vi "Shot.vi"(0 "CCD monitor in":refnum<class "CCD monitor.lvclass">, 5 "Numeric":u32, 7 "PhotoPath":path, 9 "Value":enum16{"1X1", "2X2"}(ring), 11 "error in (no error)":errorcluster) -> (4 "CCD monitor out":refnum<class "CCD monitor.lvclass">, 15 "error out":errorcluster)   [LabVIEW 2016, in "CCD monitor.lvlib" / "CCD monitor.lvclass"]
uses:
  <userlib>/Common Components/Hardware/Abstract System/Monitor/CCD monitor.lvclass
  <userlib>/Common Components/Hardware/CCD/CCD/CCD.lvclass/CCD.ctl
  <userlib>/Common Components/Hardware/Abstract System/Monitor/CCD monitor.lvclass/CCD monitor.ctl
  <userlib>/Common Components/Hardware/CCD/CCD/Read Session Out.vi
  <userlib>/Common Components/Hardware/CCD/CCD/Read New Image.vi
  <userlib>/Common Components/Hardware/CCD/CCD/CCD.lvclass
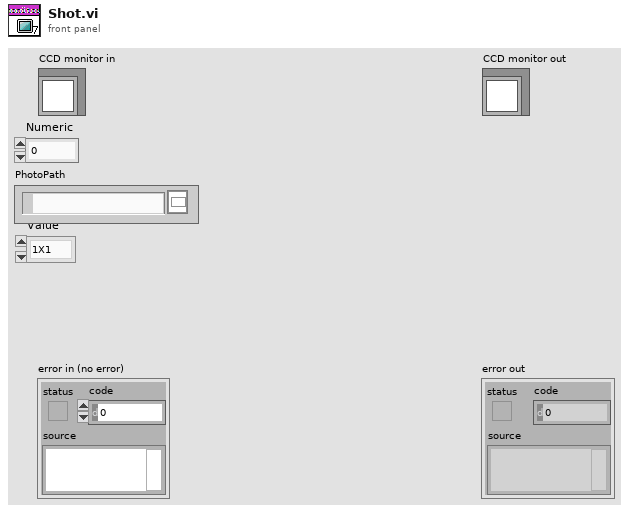
[diagram p1: front panel]
types:
  T1 = typedef "IMAQdx.ctl" = refnum<k21>
  T2 = typedef "IMAQ Image.ctl" = refnum<image>
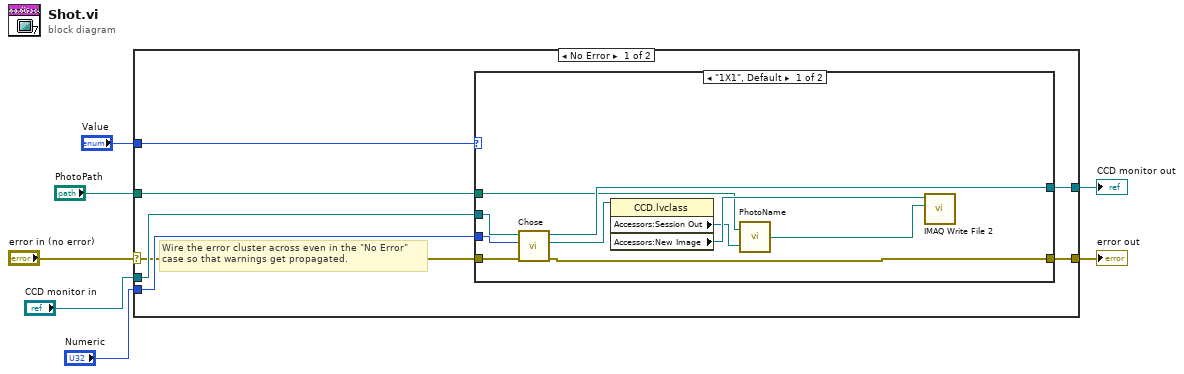
[diagram p0: block diagram]
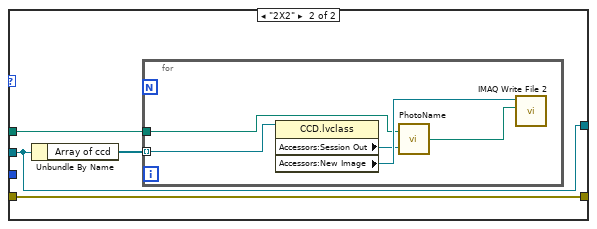
[diagram p2: hidden frame]
diagram:
  n1 = case shown="No Error" "error in (no error)" {
    selector: "error in (no error)" -> [w9 w35]
    tunnel: [w8 w35] -> w7
    tunnel: [w11 w34] -> w5
    tunnel: "CCD monitor in" -> [w12 w34]
    tunnel: "Numeric" -> [w10 _]
    tunnel: "Value" -> [w14 _]
    tunnel: "PhotoPath" -> [w13 _]
    frame No Error {
      # "Wire the error cluster across even in the \"No Error\"\ncase so that warnings get propagated."
      n2 = case shown="\"1X1\", Default" w14 {
        tunnel: w13 -> [w15 w28]
        tunnel: w12 -> [w21 w26]
        tunnel: [w19 w26] -> w11
        tunnel: w10 -> [w18 _]
        tunnel: w9 -> [w17 w25]
        tunnel: [w16 w25] -> w8
        frame "1X1", Default {
          n3 = call <userlib>:"Chose.vi"("error in (no error)"=w17, "Numeric"=w18, "CCD monitor in"=w21) -> ("error out"=w16:errorcluster, "element"=w20:refnum<class "CCD.lvclass">, "CCD monitor out"=w19:refnum<class "CCD monitor.lvclass">)  [unwired: 6 in]
          n4 = property class="CCD.lvclass"(reference=w20) -> ("Accessors:Session Out"=w23:T1, "Accessors:New Image"=w24:T2)  [unwired: 1 in, 2 out]
          n5 = call <userlib>:"PhotoName.vi"("String"=w23, "PhotoPath"=w15) -> ("path"=w22:path)
          n6 = call-poly "IMAQ Write File 2"("File Path"=w22, "Image"=w24) -> ()  [unwired: 8 in, 2 out]
        }
        frame "2X2" {
          n7 = Unbundle By Name(w26) -> ("Array of ccd"=w27:refnum<class "CCD.lvclass">[])
          n8 = for {
            tunnel: w28 -> [w30]
            tunnel: w27 -> [w29] mode=indexing
            n9 = property class="CCD.lvclass"(reference=w29) -> ("Accessors:Session Out"=w32:T1, "Accessors:New Image"=w33:T2)  [unwired: 1 in, 2 out]
            n10 = call <userlib>:"PhotoName.vi"("String"=w32, "PhotoPath"=w30) -> ("path"=w31:path)
            n11 = call-poly "IMAQ Write File 2"("File Path"=w31, "Image"=w33) -> ()  [unwired: 8 in, 2 out]
          }
        }
      }
    }
    frame Error {
    }
  }
  "error out" <- w7
  "CCD monitor out" <- w5
